vi "IC_Grab_IMAQ_Ed.vi"(4 "Error In (no error)":errorcluster, 5 "Image Dest":T1, 6 "BorderSize":i32=3, 7 "ICImagingControl In":refnum<k7>) -> (0 "Error Out":errorcluster, 1 "SampleStartTime":dbl, 2 "Image Out":T1, 3 "ICImagingControl Out":refnum<k7>)   [LabVIEW 2013]
uses:
  <vilib>/vision/Image Controls.llb/IMAQ Image.ctl
  <userlib>/IC LabVIEW Extension 2.dll
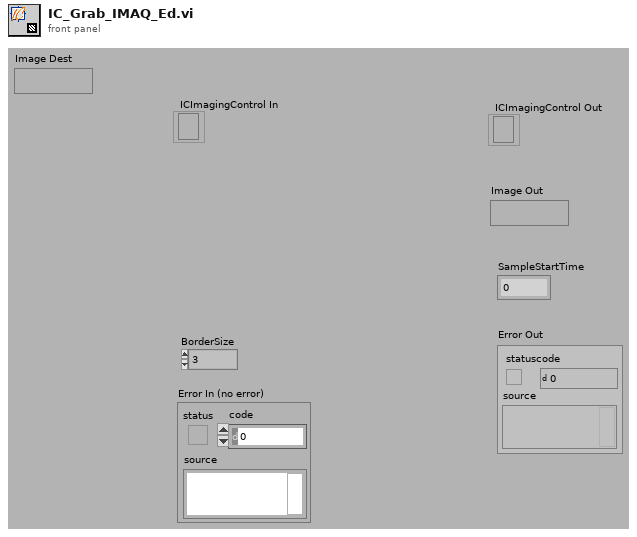
[diagram p1: front panel]
types:
  T1 = typedef "IMAQ Image.ctl" = refnum<image>
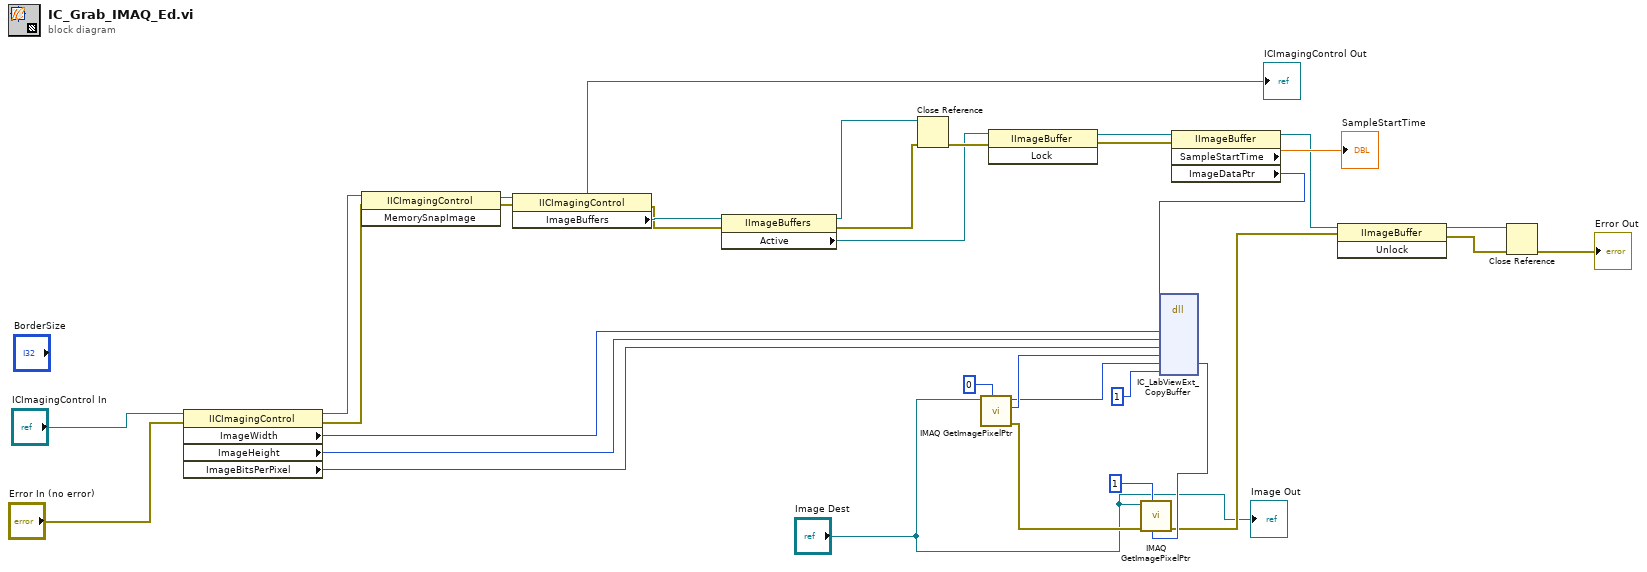
[diagram p0: block diagram]
diagram:
  n1 = property class="IICImagingControl"(reference="ICImagingControl In", error in="Error In (no error)") -> (reference out=w6:refnum<k7>, error out=w5:errorcluster, "ImageWidth"=w29:i32, "ImageHeight"=w28:i32, "ImageBitsPerPixel"=w27:i32)
  n2 = invoke class="IICImagingControl" method="MemorySnapImage"(reference=w6, error in=w5) -> (reference out=w18:refnum<k7>, error out=w4:errorcluster)  [unwired: 1 in, 1 out]
  n3 = property class="IICImagingControl"(reference=w18, error in=w4) -> (reference out=→"ICImagingControl Out":refnum<k7>, error out=w3:errorcluster, "ImageBuffers"=w21:refnum<k7>)
  n4 = property class="IImageBuffers"(reference=w21, error in=w3) -> (reference out=w7:refnum<k7>, error out=w2:errorcluster, "Active"=w8:refnum<k7>)
  n5 = Close Reference(reference=w7, error in (no error)=w2) -> (error out=w11:errorcluster)
  n6 = call "IMAQ GetImagePixelPtr"("Function"=0, "Image"="Image Dest") -> ("error out"=w31:errorcluster, "LineWidth(Pixels)"=w26:i32, "Pixel Pointer out"=w25:u64)  [unwired: 4 in, 3 out]
  n7 = invoke class="IImageBuffer" method="Lock"(reference=w8, error in=w11) -> (reference out=w9:refnum<k7>, error out=w10:errorcluster)  [unwired: 1 in, 1 out]
  n8 = property class="IImageBuffer"(reference=w9, error in=w10) -> (reference out=w13:refnum<k7>, "SampleStartTime"=→"SampleStartTime":dbl, "ImageDataPtr"=w12:i32)  [unwired: 1 out]
  n9 = dll-call lib="C:/Program Files (x86)/National Instruments/LabVIEW 2013/user.lib/IC LabVIEW Extension 2.dll" fn="IC_LabViewExt_CopyBuffer"("data"=w12, "width"=w29, "height"=w28, "bpp"=w27, "imaq_width"=w26, "imaq_ptr"=w25, "bFlip"=1) -> ("imaq_ptr"=w23:u32)  [unwired: 10 in, 2 out]
  n10 = call "IMAQ GetImagePixelPtr"("Pixel Pointer in"=w23, "Function"=1, "error in (no error)"=w31, "Image"="Image Dest") -> ("error out"=w17:errorcluster)  [unwired: 2 in, 5 out]
  n11 = invoke class="IImageBuffer" method="Unlock"(reference=w13, error in=w17) -> (reference out=w16:refnum<k7>, error out=w15:errorcluster)  [unwired: 1 in, 1 out]
  n12 = Close Reference(reference=w16, error in (no error)=w15) -> (error out=→"Error Out":errorcluster)
  "Image Out" <- "Image Dest"
